vi "Write frames.vi"(5 "frames":refnum<class "FlatSequenceFrame.lvclass">[](array[class]), 9 "FlatSequence in":refnum<class "FlatSequence.lvclass">) -> (3 "FlatSequence out":refnum<class "FlatSequence.lvclass">)   [LabVIEW 2014, in "Raspberry Pi Compatible Compiler for LabVIEW.lvlib" / "FlatSequence.lvclass"]
uses:
  FlatSequence.lvclass
  FlatSequenceFrame/FlatSequenceFrame.lvclass
  FlatSequence.lvclass/FlatSequence.ctl
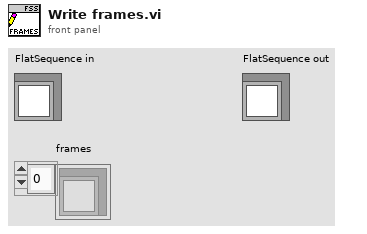
[diagram p1: front panel]
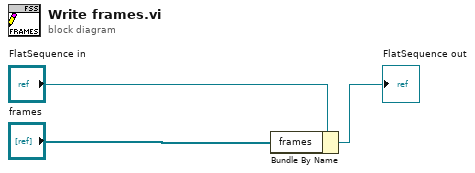
[diagram p0: block diagram]
diagram:
  n1 = Bundle By Name(cluster="FlatSequence in", "frames"="frames") -> (→"FlatSequence out":refnum<class "FlatSequence.lvclass">)
